vi "Meas End UI.vi"(8 "error in (no error)":errorcluster, 11 "UI Data in":T1) -> (0 "error out":errorcluster)   [LabVIEW 2014]
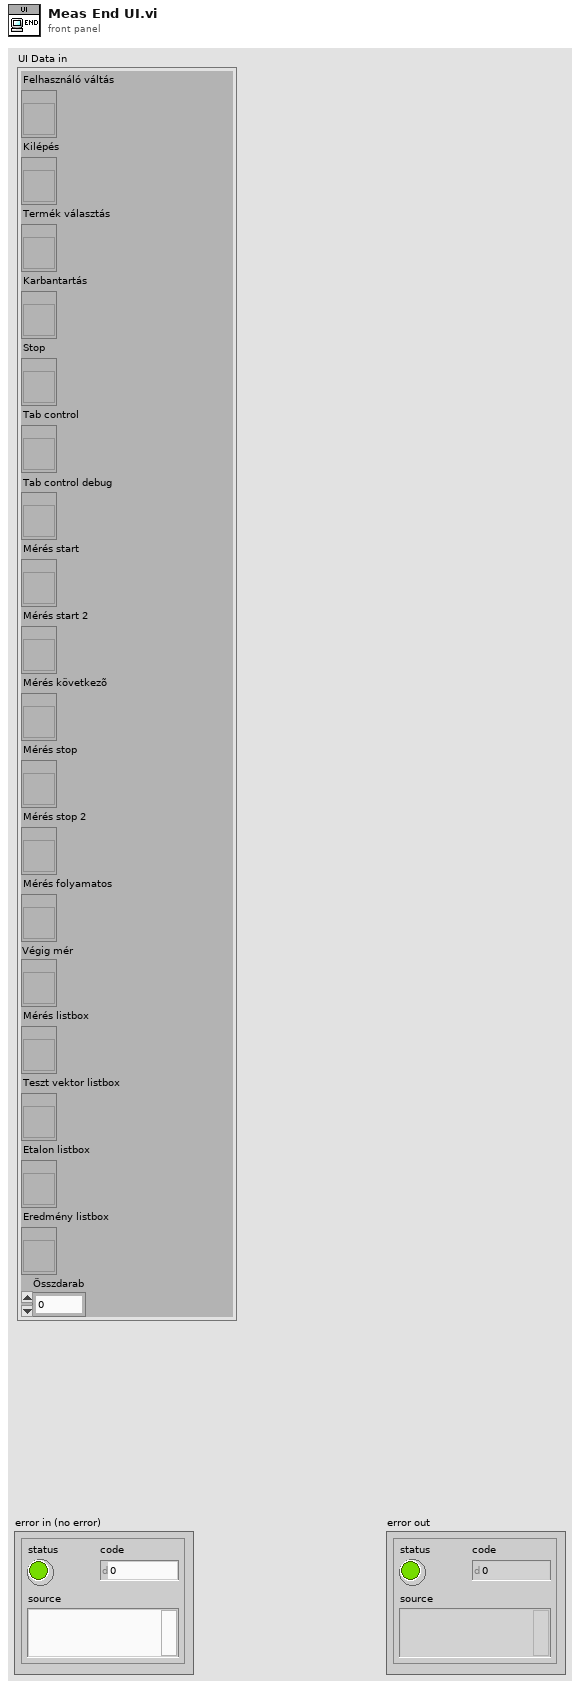
[diagram p1: front panel]
types:
  T1 = typedef "Fõképernyõ references.ctl" = cluster{"Felhasználó váltás":refnum<vi>, "Kilépés":refnum<vi>, "Termék választás":refnum<vi>, "Karbantartás":refnum<vi>, "Stop":refnum<vi>, "Tab control":refnum<vi>, "Tab control debug":refnum<vi>, "Mérés start":refnum<vi>, "Mérés start 2":refnum<vi>, "Mérés következõ":refnum<vi>, "Mérés stop":refnum<vi>, "Mérés stop 2":refnum<vi>, "Mérés folyamatos":refnum<vi>, "Végig mér":refnum<vi>, "Mérés listbox":refnum<vi>, "Teszt vektor listbox":refnum<vi>, "Etalon listbox":refnum<vi>, "Eredmény listbox":refnum<vi>, "Összdarab":i64}
  T2 = enum8{"Enabled", "Disabled", "Disabled and Grayed Out"}
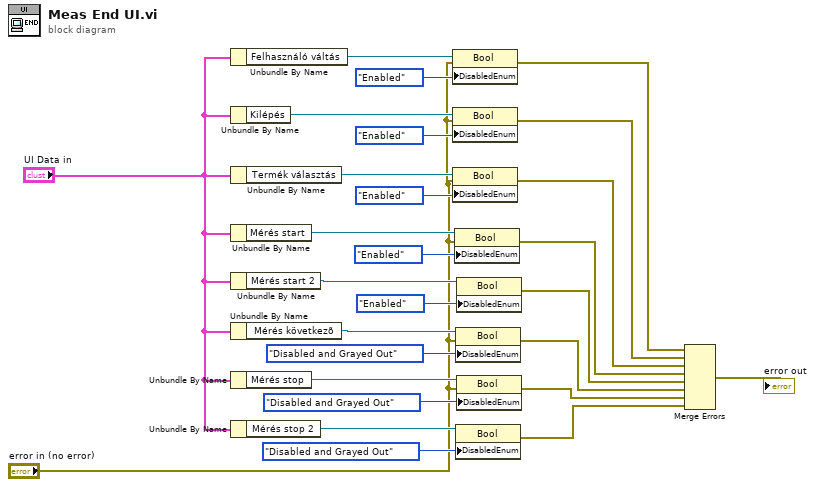
[diagram p0: block diagram]
diagram:
  n1 = Unbundle By Name("UI Data in") -> ("Felhasználó váltás"=w6:refnum<vi>)
  n2 = Unbundle By Name("UI Data in") -> ("Kilépés"=w7:refnum<vi>)
  n3 = Unbundle By Name("UI Data in") -> ("Termék választás"=w12:refnum<vi>)
  n4 = Unbundle By Name("UI Data in") -> ("Mérés start"=w23:refnum<vi>)
  n5 = Unbundle By Name("UI Data in") -> ("Mérés start 2"=w20:refnum<vi>)
  n6 = Unbundle By Name("UI Data in") -> ("Mérés következõ"=w25:refnum<vi>)
  n7 = Unbundle By Name("UI Data in") -> ("Mérés stop"=w26:refnum<vi>)
  n8 = Unbundle By Name("UI Data in") -> ("Mérés stop 2"=w15:refnum<vi>)
  n9 = property on="Property Node" class="Bool"(reference=w6, error in="error in (no error)", "DisabledEnum"=T2."Enabled" ("Disabled")) -> (error out=w1:errorcluster)  [unwired: 1 out]
  n10 = property on="Property Node" class="Bool"(reference=w7, error in="error in (no error)", "DisabledEnum"=T2."Enabled" ("Disabled")) -> (error out=w2:errorcluster)  [unwired: 1 out]
  n11 = property on="Property Node" class="Bool"(reference=w12, error in="error in (no error)", "DisabledEnum"=T2."Enabled" ("Disabled")) -> (error out=w11:errorcluster)  [unwired: 1 out]
  n12 = property on="Property Node" class="Bool"(reference=w23, error in="error in (no error)", "DisabledEnum"=T2."Enabled" ("Disabled")) -> (error out=w19:errorcluster)  [unwired: 1 out]
  n13 = property on="Property Node" class="Bool"(reference=w25, error in="error in (no error)", "DisabledEnum"=T2."Disabled and Grayed Out" ("Disabled")) -> (error out=w17:errorcluster)  [unwired: 1 out]
  n14 = property on="Property Node" class="Bool"(reference=w15, "DisabledEnum"=T2."Disabled and Grayed Out" ("Disabled")) -> (error out=w13:errorcluster)  [unwired: 1 in, 1 out]
  n15 = property on="Property Node" class="Bool"(reference=w20, "DisabledEnum"=T2."Enabled" ("Disabled")) -> (error out=w18:errorcluster)  [unwired: 1 in, 1 out]
  n16 = property on="Property Node" class="Bool"(reference=w26, error in="error in (no error)", "DisabledEnum"=T2."Disabled and Grayed Out" ("Disabled")) -> (error out=w16:errorcluster)  [unwired: 1 out]
  n17 = Merge Errors(w1, w2, w11, w19, w18, w17, w16, w13) -> (→"error out":errorcluster)
